vi "CFS-Save Cal Data.vi"(0 "Mag":dbl[](array[numeric]), 2 "Cal Stimulus":T1={"Min Freq (Hz)"=50.0, "Max Freq (Hz)"=50000.0, "Freq Step (Hz)"=50.0, "Waveform"=enum."Chirp", "Attenuation (dB)"=20.0, "Sample Rate (Hz)"=100000.0}, 5 "Phase":dbl[](array[numeric]), 7 "Frequency":dbl[](array[numeric]), 11 "error in (no error)":errorcluster, 12 "path":path) -> (6 "new file path":path, 15 "error out":errorcluster)   [LabVIEW 2015]
uses:
  Type Defs/Cal Stimulus.ctl
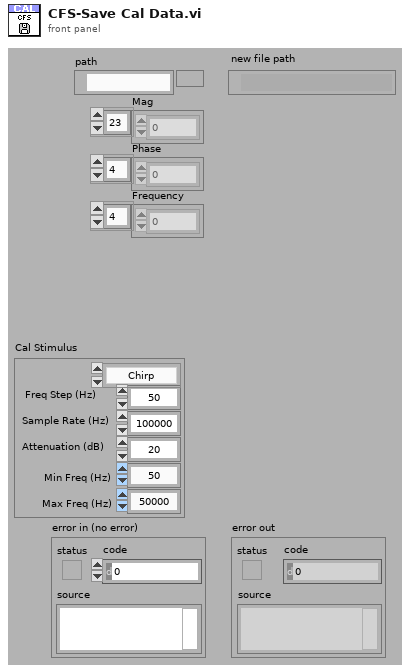
[diagram p1: front panel]
types:
  T1 = typedef "Cal Stimulus.ctl" = cluster{"Min Freq (Hz)":dbl, "Max Freq (Hz)":dbl, "Freq Step (Hz)":dbl, "Waveform":enum16{"Chirp", "Weighted"}, "Attenuation (dB)":dbl, "Sample Rate (Hz)":dbl}
  T2 = enum16{"open", "replace", "create", "open or create", "replace or create", "replace or create with confirmation"}
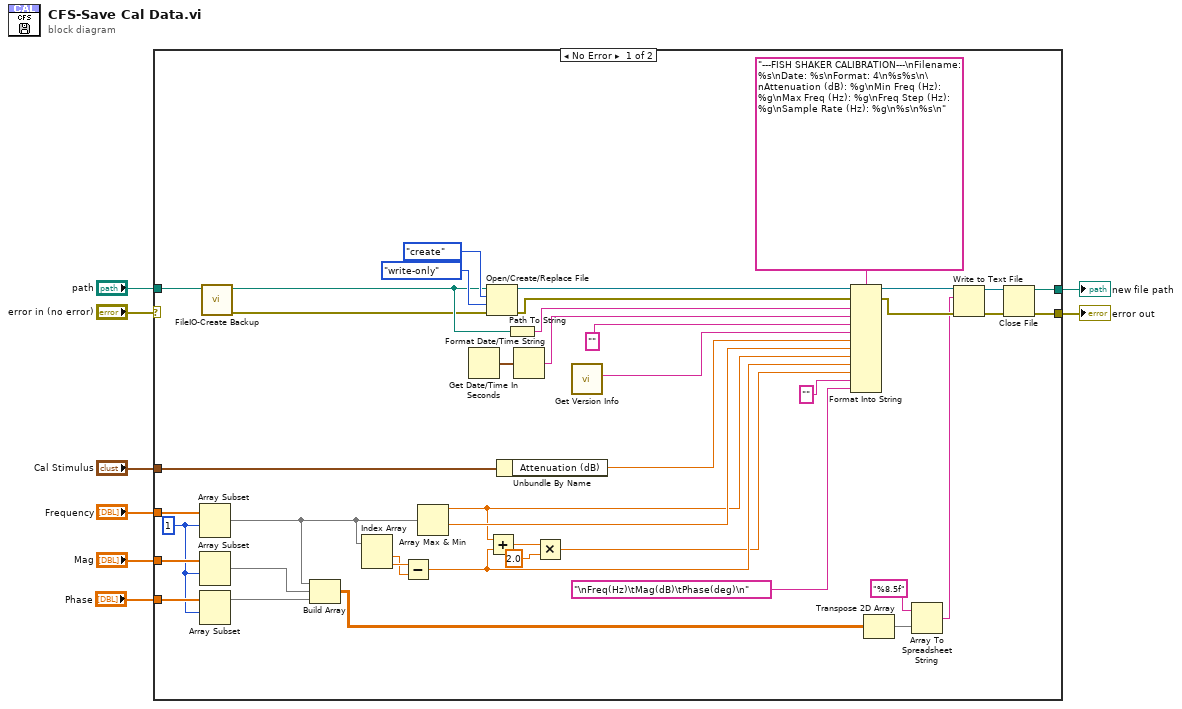
[diagram p0: block diagram]
diagram:
  n1 = case shown="No Error" "error in (no error)" {
    selector: "error in (no error)" -> [_ w51]
    tunnel: "Phase" -> [w50 _]
    tunnel: "Mag" -> [w49 _]
    tunnel: "Frequency" -> [w30 _]
    tunnel: [w36 w51] -> w5
    tunnel: "Cal Stimulus" -> [w47 _]
    tunnel: [w35 _] -> w2
    tunnel: "path" -> [w14 _]
    frame No Error {
      w27 = 1 ("index")
      n2 = Array Subset(array=w30, index=w27) -> (w25:dbl[])  [unwired: 1 in]
      n3 = Array Subset(array=w49, index=w27) -> (w29:dbl[])  [unwired: 1 in]
      n4 = Array Subset(array=w50, index=w27) -> (w28:dbl[])  [unwired: 1 in]
      n5 = call "FileIO-Create Backup.vi"("Path"=w14) -> ("error out"=w12:errorcluster, "Path (thru)"=w13:path)  [unwired: 7 in, 2 out]
      n6 = Build Array(w25, w29, w28) -> (w11:dbl[][])
      n7 = Index Array(array=w25) -> (element #1=w23:dbl, element #2=w24:dbl)  [unwired: 2 in]
      n8 = Subtract(x=w24, y=w23) -> (x-y=w21:dbl)
      n9 = Array Max & Min(array=w25) -> (max value=w22:dbl, min value=w26:dbl)  [unwired: 2 out]
      n10 = Get Date/Time In Seconds() -> (seconds since 1Jan1904=w45:timestamp)
      n11 = Open/Create/Replace File(file path (use dialog)=w13, error in=w12, operation (0:open)=T2."create", access (0:read/write)=enum16{"read/write", "read-only", "write-only"}."write-only") -> (refnum out=w34:refnum<file>, error out=w31:errorcluster)  [unwired: 2 in, 1 out]
      n12 = Add(x=w22, y=w21) -> (x+y=w20:dbl)
      n13 = Unbundle By Name(w47) -> ("Attenuation (dB)"=w15:dbl)
      n14 = Path To String(path=w13) -> (string=w46:string)
      n15 = Format Date/Time String(seconds (now)=w45) -> (date/time string=w44:string)  [unwired: 2 in]
      n16 = Multiply(x=w20, y=2.0) -> (x*y=w18:dbl)
      n17 = call "Get Version Info.vi"() -> ("Version Info"=w16:string)  [unwired: 10 in, 1 out]
      n18 = Format Into String(format string="---FISH SHAKER CALIBRATION---\nFilename: %s\nDate: %s\nFormat: 4\n%s%s\n\nAttenuation (dB): %g\nMin Freq (Hz): %g\nMax Freq (Hz): %g\nFreq Step (Hz): %g\nSample Rate (Hz): %g\n%s\n%s\n", initial string=w34, error in=w31, w46, w44, "", w16, w15, w26, w22, w21, w18, "" ("input 10"), "\nFreq(Hz)\tMag(dB)\tPhase(deg)\n" ("format string")) -> (resulting string=w41:refnum<file>, error out=w40:errorcluster)
      n19 = Transpose 2D Array(2D array=w11) -> (transposed array=w42:dbl[][])
      n20 = Array To Spreadsheet String(array=w42, 3:"%8.5f" ("format (%.3f)")) -> (spreadsheet string=w39:string)  [unwired: 1 in]
      n21 = Write to Text File(file (use dialog)=w41, text=w39, error in=w40) -> (refnum out=w37:refnum<file>, error out=w38:errorcluster)  [unwired: 1 in, 1 out]
      n22 = Close File(refnum=w37, error in=w38) -> (path=w35:path, error out=w36:errorcluster)
    }
    frame Error {
    }
  }
  "error out" <- w5
  "new file path" <- w2
